vi "SendCommand.vi"(8 "error in (no error)":errorcluster, 10 "Command string":string, 11 "InstControl in":refnum<class "InstrControl.lvclass">) -> (0 "error out":errorcluster, 3 "InstControl out":refnum<class "InstrControl.lvclass">)   [LabVIEW 2019, in "InstrControl.lvclass"]
uses:
  InstrControl.lvclass
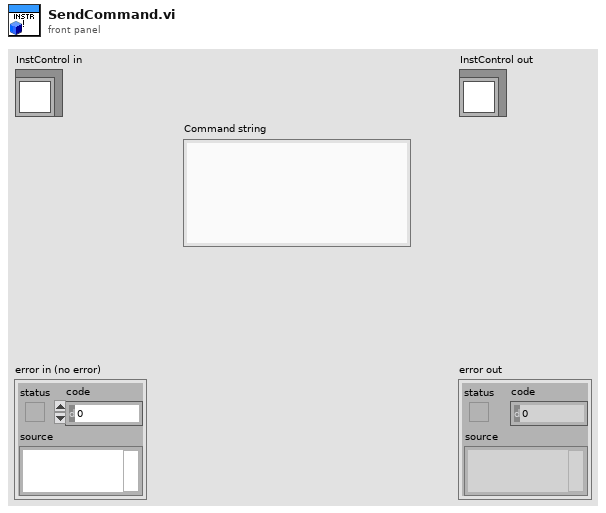
[diagram p1: front panel]
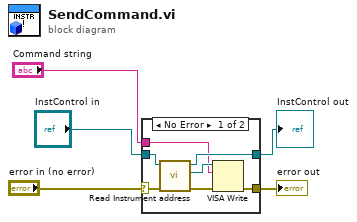
[diagram p0: block diagram]
diagram:
  n1 = case shown="No Error" "error in (no error)" {
    selector: "error in (no error)" -> [w11 w14]
    tunnel: [w6 w14] -> w4
    tunnel: [w12 w13] -> w3
    tunnel: "InstControl in" -> [w10 w13]
    tunnel: "Command string" -> [w7 _]
    frame No Error {
      n2 = call-dynamic "Read Instrument address.vi"("error in (no error)"=w11, "InstControl in"=w10) -> ("error out"=w8:errorcluster, "GPIB address"=w9:refnum<visa-resource-name>, "InstControl out"=w12:refnum<class "InstrControl.lvclass">)  [unwired: 7 in]
      n3 = VISA Write(VISA resource name=w9, write buffer=w7, error in (no error)=w8) -> (error out=w6:errorcluster)  [unwired: 2 out]
    }
    frame Error {
    }
  }
  "error out" <- w4
  "InstControl out" <- w3
